vi "Primeras pruebas.vi"() -> ()   [LabVIEW 2020]
uses:
  <vilib>/Instr/_visa.llb/VISA Open Access Mode.ctl
panel:
  out "Array":string[](array[string])
  in  "stop":bool
  out "error out":errorcluster
  out "return count":u32
  out "read buffer":string
  in  "VISA resource name":refnum<visa-resource-name>
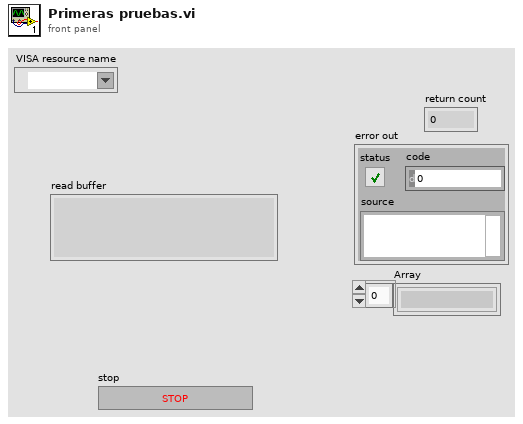
[diagram p1: front panel]
types:
  T1 = typedef "VISA Open Access Mode.ctl" = u32
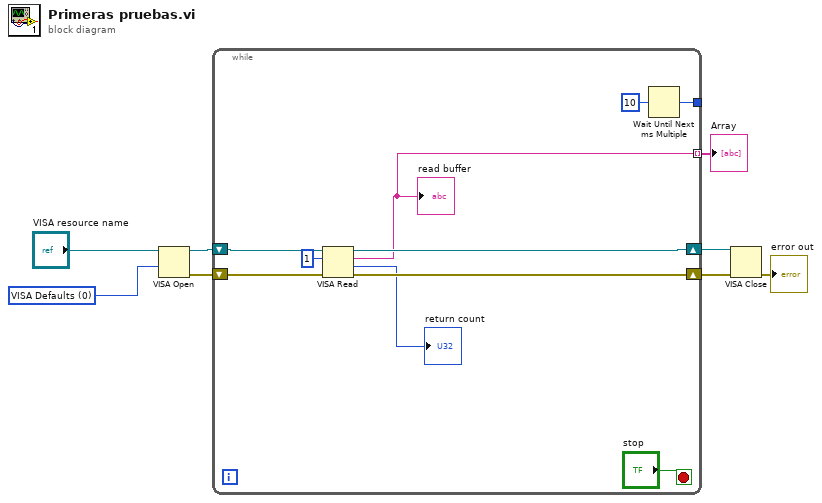
[diagram p0: block diagram]
diagram:
  w4 = T1 0 items=["VISA Defaults"=0, "Exclusive Lock"=1, "Load Configured Settings"=4] ("Access Mode")
  n1 = VISA Open(access mode=w4, VISA resource name="VISA resource name") -> (VISA resource name=w5:refnum<visa-resource-name>, error out=w3:errorcluster)  [unwired: 3 in]
  n2 = while {
    shift-right: [w18] -> w8
    shift-left: w5 -> [w16]
    shift-right: [w17] -> w7
    shift-left: w3 -> [w15]
    tunnel: [w11] -> _
    tunnel: [w9] -> w1 mode=indexing
    stop <- "stop" stop-if-true
    n3 = VISA Read(VISA resource name=w16, byte count=u32 1, error in (no error)=w15) -> (VISA resource name out=w18:refnum<visa-resource-name>, read buffer=w9:string, return count=→"return count":u32, error out=w17:errorcluster)
    "read buffer" <- w9
    n4 = Wait Until Next ms Multiple(millisecond multiple=u32 10) -> (millisecond timer value=w11:u32)
  }
  "Array" <- w1
  n5 = VISA Close(VISA resource name=w8, error in (no error)=w7) -> (error out=→"error out":errorcluster)
